vi "Logging Message Loop.vi"(8 "error in (no error)":errorcluster, 10 "Data Queue":refnum<queue>, 11 "Message Queues":T1) -> (0 "error out":errorcluster)   [LabVIEW 2021, in "Logging.lvlib"]
doc: "The message loop subVI to handle messages pertaining to logging data."
uses:
  Logging.lvlib
  support/Message Queue/All Message Queues.ctl
  support/Message Queue/Message Cluster.ctl
  controls/Acquired Data.ctl
  Logging State.ctl
  Settings/Settings.ctl
  Acquisition/Hardware Configuration.ctl
  Acquisition/Signal Type.ctl
  Interval Timer/Repeat Interval.ctl
  Interval Timer/Interval Length.ctl
  Interval Timer/Interval Token.ctl
  Logging Configuration.ctl
  Diagnostics/Diagnostics Configuration.ctl
  support/Message Queue/Enqueue Message (Single).vi
  <vilib>/Utility/error.llb/Error Cluster From Error Code.vi
  <vilib>/ErrorRing/Error Ring.xnode
  support/Message Queue/Message Queue.lvlib
  Acquisition/Acquisition.lvlib
  Settings/Settings.lvlib
  Diagnostics/Diagnostics.lvlib
  Interval Timer/Interval Timer.lvlib
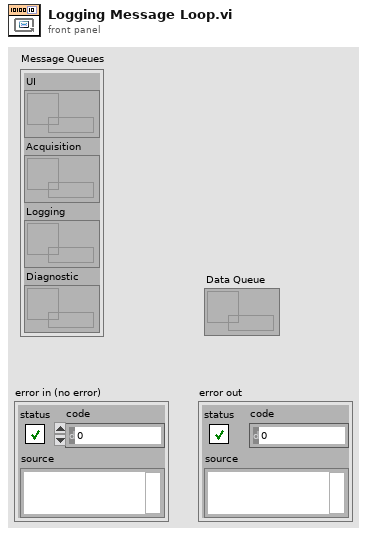
[diagram p1: front panel]
types:
  T1 = typedef "Message Queue.lvlib/All Message Queues.ctl" = cluster{"UI":refnum<queue>, "Acquisition":refnum<queue>, "Logging":refnum<queue>, "Diagnostic":refnum<queue>}
  T2 = typedef "Settings.lvlib/Settings.ctl" = cluster{"IO":T3, "Log":T8, "Debug":T9}
  T3 = typedef "Acquisition.lvlib/Hardware Configuration.ctl" = cluster{"HW Refnum <Replace Me>":string, "Signal Type <Replace Me>":T4, "Sensor Intervals":T5[], "Sensor Token":T7}
  T4 = typedef "Acquisition.lvlib/Signal Type.ctl" = enum16{"Sine Wave", "Square with Noise"}
  T5 = typedef "Interval Timer.lvlib/Repeat Interval.ctl" = cluster{"Interval":T6, "Count":i32}
  T6 = typedef "Interval Timer.lvlib/Interval Length.ctl" = enum16{"Manual control", "1 second", "10 seconds", "30 seconds", "60 seconds", "600 seconds", "1200 seconds", "3600 seconds"}
  T7 = typedef "Interval Timer.lvlib/Interval Token.ctl" = cluster{"Next reading in ms":u32, "Interval Index":i32, "Interval Occurrence":i32}
  T8 = typedef "Logging.lvlib/Logging Configuration.ctl" = cluster{"Path":path, "TDMS":refnum<k34>, "Spreadsheet":refnum<file>, "Append":bool}
  T9 = typedef "Diagnostics.lvlib/Diagnostics Configuration.ctl" = cluster{"Messages":refnum<file>}
  T10 = typedef "Logging.lvlib/Logging State.ctl" = enum16{"Idle", "Logging"}
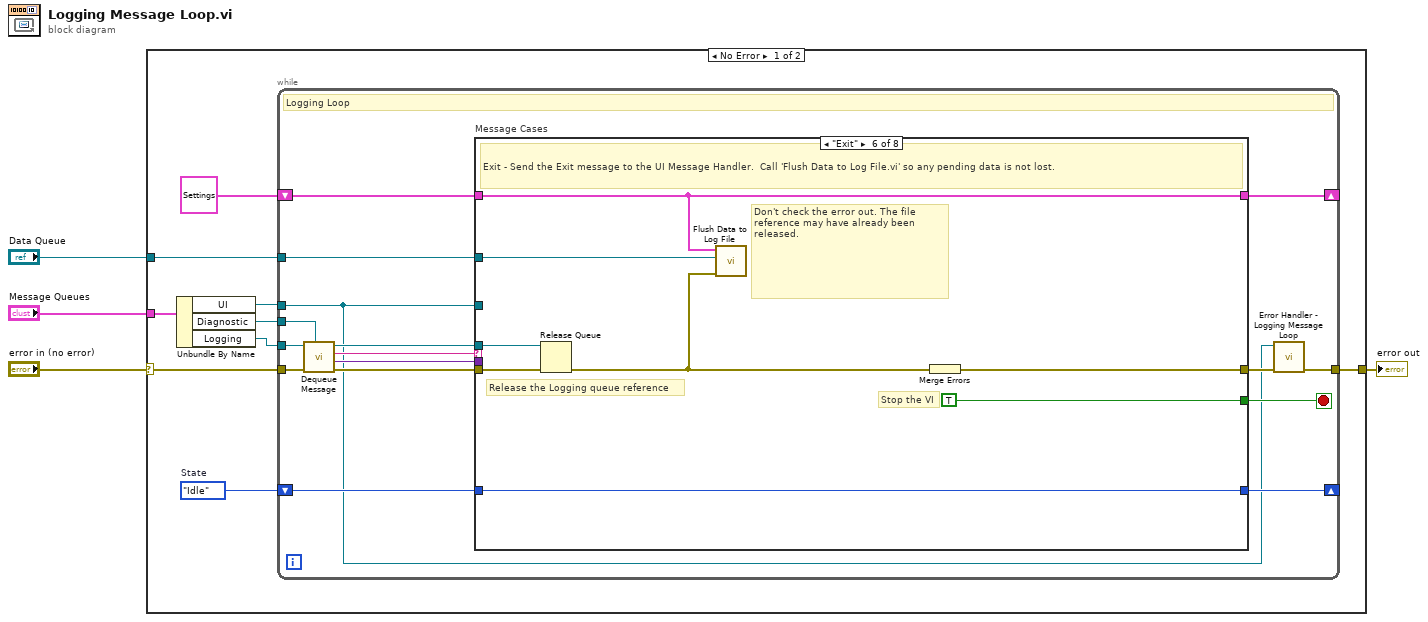
[diagram p0: block diagram]
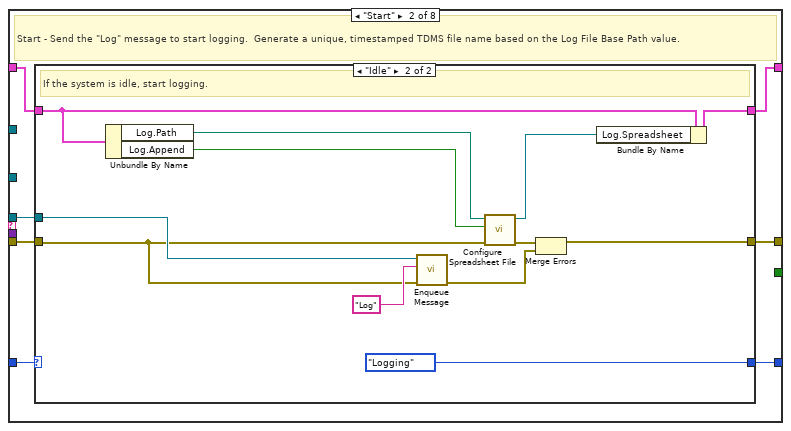
[diagram p3: hidden frame]
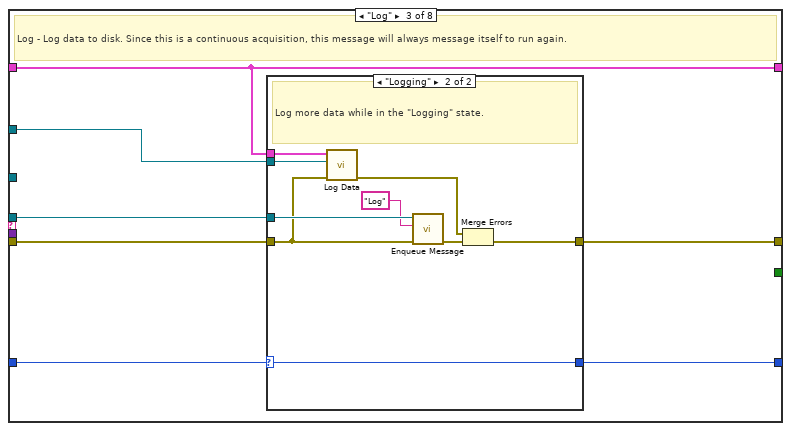
[diagram p5: hidden frame]
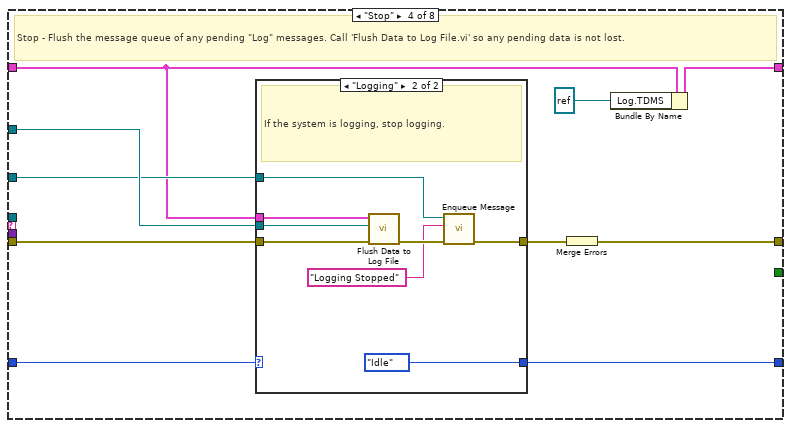
[diagram p7: hidden frame]
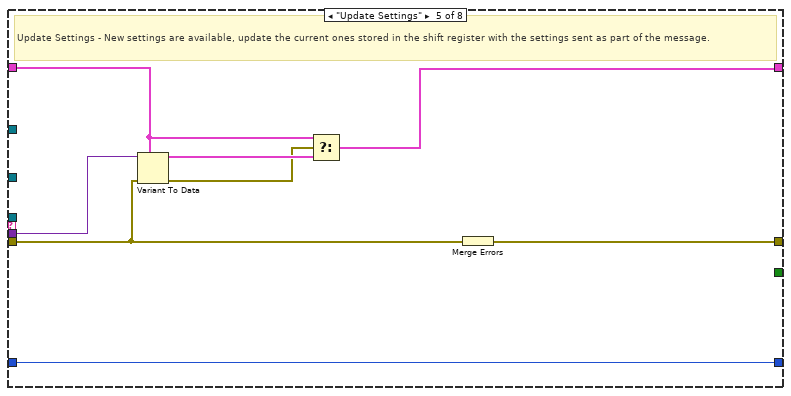
[diagram p9: hidden frame]
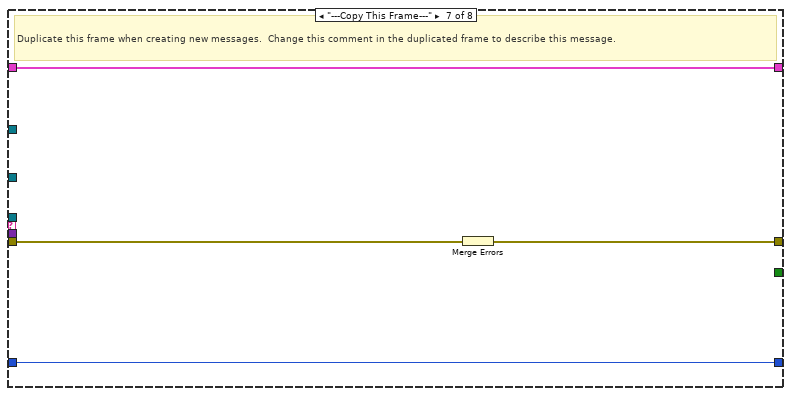
[diagram p10: hidden frame]
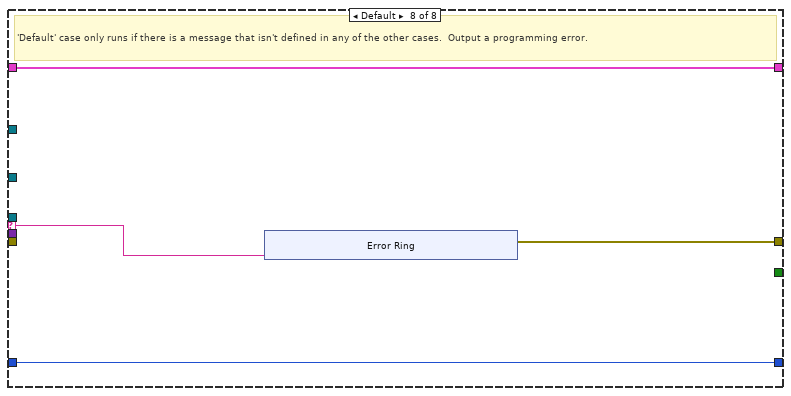
[diagram p11: hidden frame]
diagram:
  n1 = case shown="No Error" "error in (no error)" {
    selector: "error in (no error)" -> [w11 w124]
    tunnel: "Message Queues" -> [w13 _]
    tunnel: [w12 w124] -> w3
    tunnel: "Data Queue" -> [w10 _]
    frame No Error {
      w8 = Logging_State."Idle"  # State
      n2 = Unbundle By Name(w13) -> ("UI"=w9:refnum<queue>, "Diagnostic"=w5:refnum<queue>, "Logging"=w6:refnum<queue>)
      n3 = while {
        tunnel: w6 -> [w21]
        shift-right: [w28] -> _
        shift-left: T2 {"IO"={"HW Refnum <Replace Me>"="", "Signal Type <Replace Me>"=enum."Sine Wave", "Sensor Intervals"=[], "Sensor Token"={"Next reading in ms"=0, "Interval Index"=0, "Interval Occurrence"=0}}, "Log"={"Path"=path "", "TDMS"=refnum, "Spreadsheet"=refnum, "Append"=FALSE}, "Debug"={"Messages"=refnum}} ("Settings") -> [w29]
        tunnel: w9 -> [w15]
        tunnel: w10 -> [w20]
        shift-right: [w18] -> _
        shift-left: w8 -> [w19]
        tunnel: w11 -> [w26]
        tunnel: [w17] -> w12
        tunnel: w5 -> [w14]
        stop <- w27 stop-if-true
        # "Logging Loop"
        n4 = call "Dequeue Message.vi"("Diagnostics Queue"=w14, "error in (no error)"=w26, "Message Queue"=w21) -> ("error out"=w25:errorcluster, "Message Data"=w23:variant, "Message"=w24:string, "dup Message Queue"=w22:refnum<queue>)  [unwired: 5 in]
        n5 = case "Message Cases" shown="\"Exit\"" w24 {
          selector: w24 -> [_ _ _ _ _ _ _ w113]
          tunnel: w22 -> [_ w38 w60 _ _ w105 _ _]
          tunnel: w25 -> [w31 w37 w58 w77 w94 w106 w112 _]
          tunnel: [w31 w39 w61 w82 w100 w107 w110 w114] -> w16
          tunnel: w29 -> [w32 w36 w57 w73 w98 w101 w111 w116]
          tunnel: [w32 w35 w57 w80 w95 w101 w111 w116] -> w28
          tunnel: [_ _ _ _ _ TRUE _ _] -> w27
          tunnel: w23 -> [_ _ _ _ w99 _ _ _]
          tunnel: w15 -> [_ _ _ w74 _ _ _ _]
          tunnel: w20 -> [_ _ w59 w78 _ w103 _ _]
          tunnel: w19 -> [w30 w34 w56 w76 w93 w102 w109 w115]
          tunnel: [w30 w33 w55 w75 w93 w102 w109 w115] -> w18
          frame "Initialize" {
            # "Initialize - gets called when first launched. Currently a no-op."
          }
          frame "Start" {
            # "Start - Send the \"Log\" message to start logging.  Generate a unique, timestamped TDMS file name based on the Log File Base Path value."
            n6 = case shown="\"Idle\"" w34 {
              selector: w34 -> [w41 _]
              tunnel: [w40 w48] -> w39
              tunnel: w38 -> [_ w49]
              tunnel: w37 -> [w40 w47]
              tunnel: w36 -> [w42 w50]
              tunnel: [w42 w52] -> w35
              tunnel: [w41 Logging_State."Logging" ("State")] -> w33
              frame "Logging" {
                # "The system is already logging. Ignore the \"Start\" message."
              }
              frame "Idle" {
                # "If the system is idle, start logging."
                n7 = Unbundle By Name(w50) -> ("Log.Path"=w44:path, "Log.Append"=w45:bool)
                n8 = call-poly "Enqueue Message.vi"("error in (no error)"=w47, "Message"="Log", "Message Queue"=w49) -> ("error out"=w53:errorcluster)  [unwired: 7 in, 1 out]
                n9 = call "Configure Spreadsheet File.vi"("error in"=w47, "Append data?"=w45, "file path"=w44) -> ("error out"=w46:errorcluster, "file reference"=w43:refnum<file>)  [unwired: 7 in]
                n10 = Merge Errors(w46, w53) -> (w48:errorcluster)
                n11 = Bundle By Name(cluster=w50, "Log.Spreadsheet"=w43) -> (w52:T2)
              }
            }
          }
          frame "Log" {
            # "Log - Log data to disk. Since this is a continuous acquisition, this message will always message itself to run again."
            n12 = case shown="\"Logging\"" w56 {
              selector: w56 -> [w63 w65]
              tunnel: [w62 w72] -> w61
              tunnel: w60 -> [_ w70]
              tunnel: w59 -> [_ w69]
              tunnel: w58 -> [w62 w64]
              tunnel: w57 -> [_ w66]
              tunnel: [w63 w65] -> w55
              frame "Idle" {
                # "Ignore \"Log\" messages when the logging is idle."
              }
              frame "Logging" {
                # "Log more data while in the \"Logging\" state."
                n13 = call "Log Data.vi"("error in (no error)"=w64, "Data Queue"=w69, "Settings"=w66) -> ("error out"=w68:errorcluster)  [unwired: 8 in]
                n14 = call-poly "Enqueue Message.vi"("error in (no error)"=w64, "Message"="Log", "Message Queue"=w70) -> ("error out"=w71:errorcluster)  [unwired: 7 in, 1 out]
                n15 = Merge Errors(w68, w71) -> (w72:errorcluster)
              }
            }
          }
          frame "Stop" {
            # "Stop - Flush the message queue of any pending \"Log\" messages. Call 'Flush Data to Log File.vi' so any pending data is not lost."
            n16 = case shown="\"Logging\"" w76 {
              selector: w76 -> [w83 _]
              tunnel: [w84 w87] -> w81
              tunnel: w78 -> [_ w91]
              tunnel: w73 -> [_ w90]
              tunnel: w77 -> [w84 w89]
              tunnel: [w83 Logging_State."Idle" ("State")] -> w75
              tunnel: w74 -> [_ w86]
              frame "Idle" {
                # "The system is already idle. Ignore the \"Stop\" message."
              }
              frame "Logging" {
                # "If the system is logging, stop logging."
                n17 = call "Flush Data to Log File.vi"("error in (no error)"=w89, "Data Queue"=w91, "Settings"=w90) -> ("error out"=w92:errorcluster)  [unwired: 8 in]
                n18 = call-poly "Enqueue Message.vi"("error in (no error)"=w92, "Message"="Logging Stopped", "Message Queue"=w86) -> ("error out"=w87:errorcluster)  [unwired: 7 in, 1 out]
              }
            }
            n19 = Merge Errors(w81) -> (w82:errorcluster)
            n20 = Bundle By Name(cluster=w73, "Log.TDMS"=refnum<k34> refnum ("TDMS File Reference")) -> (w80:T2)
          }
          frame "Update Settings" {
            # "Update Settings - New settings are available, update the current ones stored in the shift register with the settings sent as part of the message."
            n21 = Variant To Data(error in=w94, type=w98, Variant=w99) -> (data=w97:T2, error out=w96:errorcluster)
            n22 = Select(t=w98, s=w96, f=w97) -> (s? t:f=w95:T2)
            n23 = Merge Errors(w94) -> (w100:errorcluster)
          }
          frame "Exit" {
            # "Don't check the error out. The file reference may have already been released."
            # "Release the Logging queue reference"
            # "Stop the VI"
            # "Exit - Send the Exit message to the UI Message Handler.  Call 'Flush Data to Log File.vi' so any pending data is not lost."
            n24 = Release Queue(queue=w105, error in (no error)=w106) -> (error out=w104:errorcluster)  [unwired: 1 in, 2 out]
            n25 = call "Flush Data to Log File.vi"("error in (no error)"=w104, "Data Queue"=w103, "Settings"=w101) -> ()  [unwired: 8 in, 1 out]
            n26 = Merge Errors(w104) -> (w107:errorcluster)
          }
          frame "---Copy This Frame---" {
            # "Duplicate this frame when creating new messages.  Change this comment in the duplicated frame to describe this message."
            n27 = Merge Errors(w112) -> (w110:errorcluster)
          }
          frame Default {
            # "'Default' case only runs if there is a message that isn't defined in any of the other cases.  Output a programming error."
            n28 = xnode "Error Ring"("parameter 0"=w113) -> ("error out"=w114:errorcluster)
          }
        }
        n29 = call "Error Handler - Logging Message Loop.vi"("error in (no error)"=w16, "Message Queue"=w15) -> ("dup error in"=w17:errorcluster)  [unwired: 8 in, 1 out]
      }
    }
    frame Error {
    }
  }
  "error out" <- w3
